vi "laneleftright4_2_1.vi"() -> (2 "Coeff right":dbl[](array[numeric]), 3 "Coeff left":dbl[](array[numeric]))   [LabVIEW 2015]
uses:
  <vilib>/Analysis/polynomials.llb/Remove Zero Threshold Type.ctl
  G_SEN.vi
  <vilib>/Analysis/1siggen.llb/Ramp Pattern by Delta.vi
  G_LCM.vi
  <vilib>/Analysis/polynomials.llb/1D Polynomial Evaluation (DBL).vi
  <vilib>/Analysis/polynomials.llb/Remove Zero Coefficients (DBL).vi
  G_ALL.vi
  <vilib>/Analysis/NI_AALPro.lvlib
  <vilib>/Analysis/NI_AALBase.lvlib
  <vilib>/gmath/NI_Gmath.lvlib
panel:
  out "stop_shift":dbl
  in  "y 4":dbl
  in  "y 3":dbl
  out "f":dbl
  out "x0, y0, z0 2":dbl[](array[numeric]) format="%.2f"
  out "r":dbl format="%.2f"
  in  "threshold":dbl
  out "y 2":dbl[](array[numeric])
  out "x 2":dbl[](array[numeric])
  out "w 2":dbl[](array[numeric])
  out "lane_right_pt":dbl[][](array[numeric])
  in  "x_gain":dbl=1.0 min=-1.0 max=1.0
  in  "y_gain":dbl=1.0 min=-1.0 max=1.0
  out "map_track 2":dbl[][](array[numeric])
  in  "d_safe":dbl=1.1 format="%#_13g"
  out "map_track":dbl[][](array[numeric])
  out "lane_left_pt":dbl[][](array[numeric])
  out "x_shift":dbl format="%#_13g"
  out "y_shift":dbl format="%#_13g"
  in  "lane_gain":dbl=0.7 min=-1.0 max=1.0
  out "Lane_C_M":dbl[](array[numeric])=[0.8601491478953653, 0.8717844136967624, 0.882947592858927, 0.8936326403234123, 0.9038337699485205, 0.9135454576426009, 0.9227624443554423, 0.9314797389261423, 0.9396926207859084, 0.9473966425143293, 0.9545876322477319, 0.9612616959383189, 0.9674152194628639, 0.9730448705798238, 0.9781476007338057, 0.9827206467064133, 0.9867615321125792, 0.9902680687415704, 0.993238357741943, 0.9956707906498045, 0.9975640502598242, 0.9989171113385246, 0.9997292411794617, 1.0, 0.9997292411794617, 0.9989171113385246, 0.9975640502598242, 0.9956707906498045, 0.993238357741943, 0.9902680687415704, 0.9867615321125792, 0.9827206467064133]
  out "ratio(-1:left1:right)":dbl
  out "NaN/Path/Refnum?":bool
  out "Rleft":dbl
  out "Rright":dbl
  in  "poly":i32=2 min=1 max=5 step=1
  out "Coeff stop":dbl[](array[numeric])
  out "y_end":dbl[](array[numeric])=[0.8601491478953653, 0.8717844136967624, 0.882947592858927, 0.8936326403234123, 0.9038337699485205, 0.9135454576426009, 0.9227624443554423, 0.9314797389261423, 0.9396926207859084, 0.9473966425143293, 0.9545876322477319, 0.9612616959383189, 0.9674152194628639, 0.9730448705798238, 0.9781476007338057, 0.9827206467064133, 0.9867615321125792, 0.9902680687415704, 0.993238357741943, 0.9956707906498045, 0.9975640502598242, 0.9989171113385246, 0.9997292411794617, 1.0, 0.9997292411794617, 0.9989171113385246, 0.9975640502598242, 0.9956707906498045, 0.993238357741943, 0.9902680687415704, 0.9867615321125792, 0.9827206467064133]
  in  "iter":i32=7
  out "Waveform Graph":dbl[](graph)
  out "w":dbl[](array[numeric])
  out "XY Graph 4":cluster{"Y":dbl[], "Y":dbl[]}[](graph)=[{"Y"=array[3210 elements], "Y"=array[3210 elements]}, {"Y"=[-0.0, 0.001154394197769193, 0.004617650635850623, 0.010389990872226917, 0.018471784248973222, 0.02886354801042046, 0.041565947468740205, 0.056579796217107514, 0.0739060563904701, 0.0935458389742223, 0.11550040416098284, 0.13977116175580306, 0.16635967162997645, 0.19526764422393228, 0.2264969410994837, 0.26004957554195585, 0.2959277132125635, 0.3341336728515216, 0.374669927032528, 0.417539102969144, 0.4627439833735707, 0.5102875073687159, 0.560172771454063, 0.6124030305261954, 0.6669816989546717, 0.7239123517142048, 0.7831987255740245, 0.8448447203451934, 0.9088544001870815, 0.975231994973953, 1.0439819017227023, 1.1151086860829622, 1.1886170838907617, 1.2645120027869723, 1.342798523901962, 1.42348190360768, 1.5065675753387922, 1.592061151484188, 1.6799684253507792, 1.770295373200753, 1.8630481563645134, 1.9582331234307588, 2.0558568125157564, 2.1559259536137603, 2.258447471030621], "Y"=[0.0, 0.5, 1.0, 1.5, 2.0, 2.5, 3.0, 3.5, 4.0, 4.5, 5.0, 5.5, 6.0, 6.5, 7.0, 7.5, 8.0, 8.5, 9.0, 9.5, 10.0, 10.5, 11.0, 11.5, 12.0, 12.5, 13.0, 13.5, 14.0, 14.5, 15.0, 15.5, 16.0, 16.5, 17.0, 17.5, 18.0, 18.5, 19.0, 19.5, 20.0, 20.5, 21.0, 21.5, 22.0]}, {"Y"=[0.362252581831572], "Y"=[-0.8199241909738847]}, {"Y"=array[210 elements], "Y"=array[210 elements]}, {"Y"=[-0.925, -0.925, -0.925, -0.6775, -0.6775, -0.925, -0.925, -0.925, -0.925, -0.6775, -0.6775, -0.925, -0.925, -0.925, 0.9025, 0.9025, 0.9025, 0.6775, 0.6775, 0.9025, 0.9025, 0.9025, 0.9025, 0.6775, 0.6775, 0.9025, 0.9025, 0.9025, -0.925], "Y"=[-0.75, -0.224, 0.224, 0.224, -0.224, -0.224, 0.224, 2.415, 2.885, 2.885, 2.415, 2.415, 2.885, 3.5, 3.5, 2.885, 2.415, 2.415, 2.885, 2.885, 2.415, 0.224, -0.224, -0.224, 0.224, 0.224, -0.224, -0.75, -0.75]}, {"Y"=[0.171875, 0.15377271904051304, 0.1346290179491043, 0.11445423440635205, 0.09325870609283447, 0.07105277068912982, 0.04784676587581635, 0.02365102933347224, -0.0015241012573242174, -0.02766828821599482, -0.05477119386196136, -0.08282248051464558, -0.11181181049346922, -0.14172884611785413, -0.17256324970722198, -0.20430468358099463, -0.23694281005859374, -0.27046729145944115, -0.30486779010295867, -0.340133968308568, -0.3762554883956909, -0.41322201268374914, -0.4510232034921646, -0.4896487231403589], "Y"=[0.0, 0.5, 1.0, 1.5, 2.0, 2.5, 3.0, 3.5, 4.0, 4.5, 5.0, 5.5, 6.0, 6.5, 7.0, 7.5, 8.0, 8.5, 9.0, 9.5, 10.0, 10.5, 11.0, 11.5]}, {"Y"=[1.796875, 1.778772719040513, 1.7596290179491043, 1.739454234406352, 1.7182587060928345, 1.6960527706891297, 1.6728467658758164, 1.6486510293334722, 1.6234758987426758, 1.5973317117840051, 1.5702288061380387, 1.5421775194853544, 1.513188189506531, 1.483271153882146, 1.452436750292778, 1.4206953164190055, 1.3880571899414063, 1.354532708540559, 1.3201322098970414, 1.284866031691432, 1.248744511604309, 1.2117779873162509, 1.1739767965078354, 1.135351276859641, 1.0959117660522462, 1.0556686017662287, 1.014632121682167, 0.9728126634806396, 0.9302205648422242, 0.8868661634474992], "Y"=[0.0, 0.5, 1.0, 1.5, 2.0, 2.5, 3.0, 3.5, 4.0, 4.5, 5.0, 5.5, 6.0, 6.5, 7.0, 7.5, 8.0, 8.5, 9.0, 9.5, 10.0, 10.5, 11.0, 11.5, 12.0, 12.5, 13.0, 13.5, 14.0, 14.5]}, {"Y"=[-1.453125, -1.471227280959487, -1.4903709820508957, -1.510545765593648, -1.5317412939071655, -1.5539472293108703, -1.5771532341241836, -1.6013489706665278, -1.6265241012573242, -1.6526682882159949, -1.6797711938619613, -1.7078224805146456, -1.736811810493469, -1.766728846117854, -1.797563249707222, -1.8293046835809945, -1.8619428100585937, -1.895467291459441, -1.9298677901029586], "Y"=[0.0, 0.5, 1.0, 1.5, 2.0, 2.5, 3.0, 3.5, 4.0, 4.5, 5.0, 5.5, 6.0, 6.5, 7.0, 7.5, 8.0, 8.5, 9.0]}, {"Y"=[0.171875, 0.2568230007600336, 0.3384052130063493, 0.44574342526006827, 0.5205081969556753, 0.5917680690742042, 0.659409530134929, 0.7229937549325056, 0.7835496148685115, 0.8405449546633443, 0.9258576868463875], "Y"=[-20.239964538708662, -19.725637940364884, -19.211158961966362, -18.6998967366845, -18.19022720070031, -17.681887266143153, -17.17615515566314, -16.67683575591291, -16.176265245349786, -15.679082775270938, -15.183754484614711]}, {"Y"=[7.134647485270904], "Y"=[38.71960961082238]}, {"Y"=array[980 elements], "Y"=array[980 elements]}, {"Y"=[], "Y"=[]}]
  out "y":dbl[](array[numeric])
  out "x":dbl[](array[numeric])
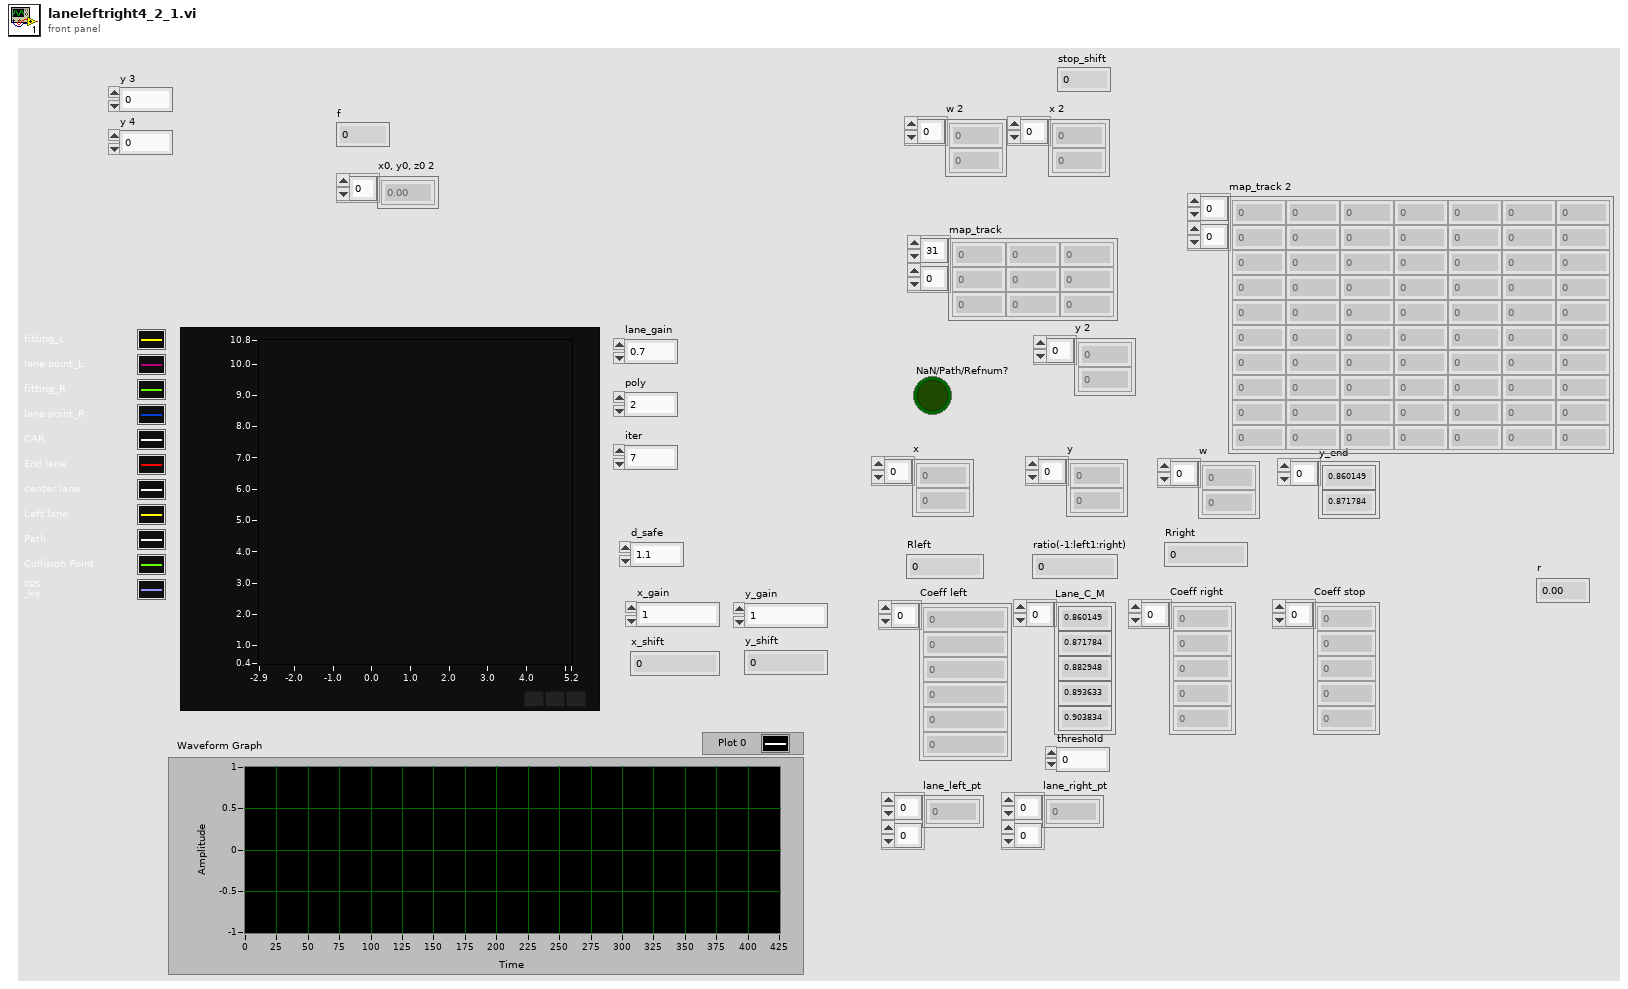
[diagram p1: front panel]
types:
  T1 = cluster{"hash":i64, "sys time":i64, "size":i64, "x":dbl[], "y":dbl[], "point_flag":i32[]}
  T2 = cluster{"delta":bool, "Rotational position":dbl, "Rotational position":dbl}[]
  T3 = typedef "NI_AALPro.lvlib/Remove Zero Threshold Type.ctl" = u16
  T4 = cluster{"C_Wheel base":dbl, "ratio_steer":dbl, "Overall width":dbl, "af":dbl, "turn radius":dbl, "eval":dbl, "ap":dbl, "an":dbl, "Vmax":dbl, "mu":dbl, "Vlast":dbl}
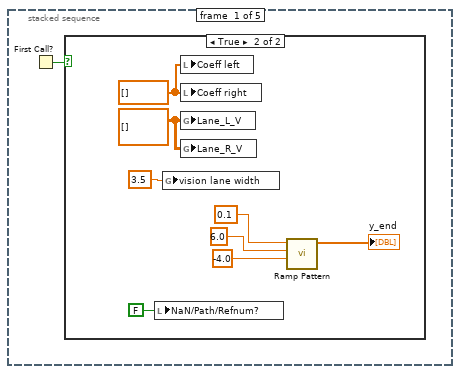
[diagram p2: hidden frame]
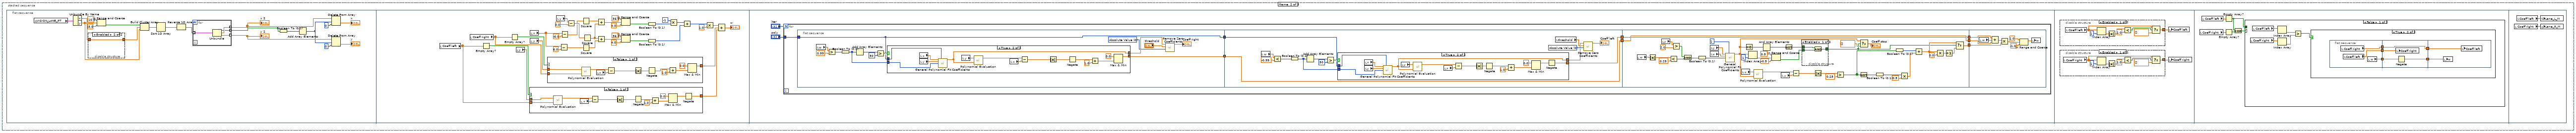
[diagram p4: hidden frame]
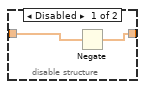
[diagram p5: hidden frame]
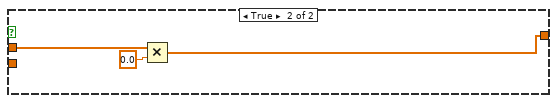
[diagram p6: hidden frame]
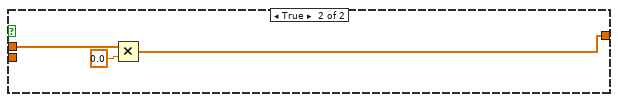
[diagram p7: hidden frame]
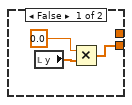
[diagram p8: hidden frame]
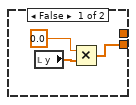
[diagram p9: hidden frame]
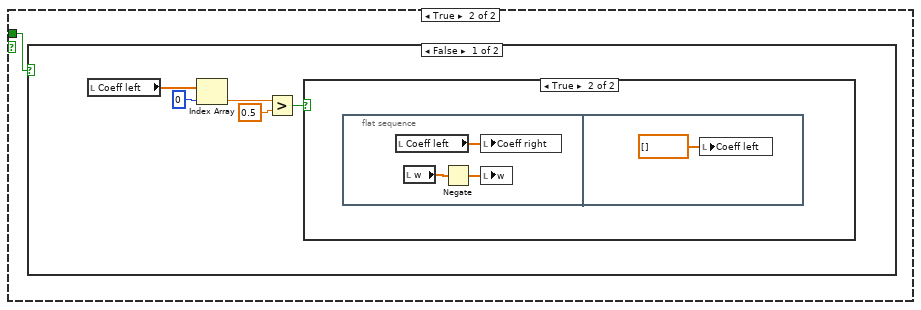
[diagram p14: hidden frame]
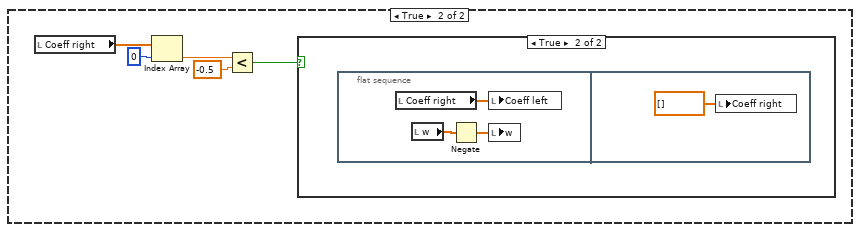
[diagram p16: hidden frame]
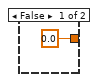
[diagram p19: hidden frame]
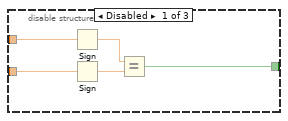
[diagram p20: hidden frame]
diagram:
  n1 = stacked-sequence {
    frame #0 {
      n2 = First Call?() -> (First Call?: T/F=w1:bool)
      n3 = case shown="True" w1 {
        frame False {
        }
        frame True {
          w2 = dbl[] [] ("Coeff left")
          w4 = dbl[][] [] ("Lane_R_V")
          n4 = local write "NaN/Path/Refnum?"(FALSE ("NaN/Path/Refnum?")) -> ()
          n5 = global write "G_SEN.vi" "vision lane width"(3.5 ("vision lane width")) -> ()
          n6 = local write "Coeff left"(w2) -> ()
          n7 = local write "Coeff right"(w2) -> ()
          n8 = global write "G_SEN.vi" "Lane_L_V"(w4) -> ()
          n9 = global write "G_SEN.vi" "Lane_R_V"(w4) -> ()
          n10 = call-poly <vilib>:"Ramp Pattern.vi"("start"=-4.0, "end"=6.0, "delta"=0.1) -> ("Ramp Pattern"=→"y_end":dbl[])  [unwired: 6 in, 2 out]
        }
      }
    }
    frame #1 {
      n11 = flat-sequence {
        frame #0 {
          n12 = global read "G_LCM.vi" "VISION_LANE_PT"() -> (w12:T1)
          n13 = Unbundle By Name(w12) -> ("x"=w27:dbl[], "y"=w21:dbl[])
          n14 = disable-structure shown="Enabled" {
            disable-tunnel: w27 -> [w30 w31]
            disable-tunnel: [w29 w31] -> w28
            frame Disabled {
              n15 = Negate(x=w30) -> (-x=w29:dbl[])
            }
            frame Enabled {
            }
          }
          n16 = In Range and Coerce(upper limit=10.0 ("delta"), x=w21, lower limit=-3.0) -> (In Range?=w19:bool[])  [unwired: 1 out]
          n17 = Build Cluster Array(w19, w28, w21) -> (w17:T2)
          n18 = Sort 1D Array(array=w17) -> (sorted array=w18:T2)
          n19 = Reverse 1D Array(array=w18) -> (reversed array=w14:T2)
          n20 = for {
            tunnel: w14 -> [w35] mode=indexing
            tunnel: [w34] -> w11 mode=indexing
            tunnel: [w33] -> w10 mode=indexing
            tunnel: [w32] -> w22 mode=indexing
            n21 = Unbundle(w35) -> ("delta"=w32:bool, "Rotational position"=w34:dbl, "Rotational position"=w33:dbl)
          }
          "x 2" <- w11
          "y 2" <- w10
          n22 = Boolean To (0,1)(Boolean=w22) -> (0, 1=w15:i16[])
          n23 = Add Array Elements(numeric array=w15) -> (sum=w23:i16)
          n24 = Delete From Array(array=w11, length=w23, index=0) -> (deleted portion=→"x":dbl[])  [unwired: 1 out]
          n25 = Delete From Array(array=w10, length=w23, index=0) -> (deleted portion=→"y":dbl[])  [unwired: 1 out]
        }
        frame #1 {
          n26 = local read "Coeff left"() -> (w67:dbl[])
          n27 = local read "Coeff right"() -> (w66:dbl[])
          n28 = Empty Array?(array=w67) -> (empty?=w68:bool)
          n29 = Empty Array?(array=w66) -> (empty?=w69:bool)
          n30 = local read "y"() -> (w64:dbl[])
          n31 = case shown="False" w68 {
            tunnel: w64 -> [w90 w98]
            tunnel: w67 -> [w87 _]
            tunnel: [w85 w97] -> w65
            frame False {
              n32 = call-poly <vilib>:"Polynomial Evaluation.vi"("P(x)"=w87, "A"=w90) -> ("P(A)"=w89:dbl[])  [unwired: 1 out]
              n33 = local read "x"() -> (w88:dbl[])
              n34 = Subtract(x=w89, y=w88) -> (x-y=w94:dbl[])
              n35 = Absolute Value(x=w94) -> (abs(x)=w93:dbl[])
              n36 = Negate(x=w93) -> (-x=w92:dbl[])
              n37 = Add(x=w92, y=1.0) -> (x+y=w96:dbl[])
              n38 = Max & Min(x=0.0, y=w96) -> (max(x,y)=w86:dbl[])  [unwired: 1 out]
              n39 = Negate(x=w86) -> (-x=w85:dbl[])
            }
            frame True {
              n40 = Multiply(x=w98, y=0.0) -> (x*y=w97:dbl[])
            }
          }
          n41 = local read "x"() -> (w36:dbl[])
          n42 = local read "y"() -> (w70:dbl[])
          n43 = case shown="False" w69 {
            tunnel: [w79 w82] -> w62
            tunnel: w66 -> [w78 _]
            tunnel: w70 -> [w71 w83]
            frame False {
              n44 = call-poly <vilib>:"Polynomial Evaluation.vi"("P(x)"=w78, "A"=w71) -> ("P(A)"=w76:dbl[])  [unwired: 1 out]
              n45 = local read "x"() -> (w77:dbl[])
              n46 = Subtract(x=w76, y=w77) -> (x-y=w72:dbl[])
              n47 = Absolute Value(x=w72) -> (abs(x)=w73:dbl[])
              n48 = Negate(x=w73) -> (-x=w74:dbl[])
              n49 = Add(x=w74, y=1.0) -> (x+y=w80:dbl[])
              n50 = Max & Min(x=0.0, y=w80) -> (max(x,y)=w79:dbl[])  [unwired: 1 out]
            }
            frame True {
              n51 = Multiply(x=w83, y=0.0) -> (x*y=w82:dbl[])
            }
          }
          n52 = local read "y"() -> (w37:dbl[])
          n53 = Subtract(x=w36, y=6.0) -> (x-y=w40:dbl[])
          n54 = Subtract(x=w36, y=-6.0) -> (x-y=w42:dbl[])
          n55 = Subtract(x=w37, y=0.0) -> (x-y=w49:dbl[])
          n56 = Square(x=w42) -> (x^2=w41:dbl[])
          n57 = Square(x=w40) -> (x^2=w50:dbl[])
          n58 = Square(x=w49) -> (x^2=w51:dbl[])
          n59 = Add(x=w41, y=w51) -> (x+y=w57:dbl[])
          n60 = Add(x=w51, y=w50) -> (x+y=w52:dbl[])
          n61 = In Range and Coerce(upper limit=36.0, x=w57, lower limit=4.0) -> (In Range?=w59:bool[])  [unwired: 1 out]
          n62 = In Range and Coerce(upper limit=36.0, x=w52, lower limit=4.0) -> (In Range?=w58:bool[])  [unwired: 1 out]
          n63 = Boolean To (0,1)(Boolean=w59) -> (0, 1=w60:i16[])
          n64 = Boolean To (0,1)(Boolean=w58) -> (0, 1=w61:i16[])
          n65 = Multiply(x=i16 -1, y=w60) -> (x*y=w45:i16[])
          n66 = Add(x=w45, y=w61) -> (x+y=w47:i16[])
          n67 = Multiply(x=w47, y=1.0 ("element")) -> (x*y=w63:dbl[])
          n68 = Compound Arithmetic op=ADD(w63, w62, w65) -> (→"w":dbl[])
        }
        frame #2 {
          n69 = for {
            N: "iter" -> [_]
            tunnel: "poly" -> [w103]
            n70 = flat-sequence {
              tunnel: [w120] -> w109
              tunnel: w103 -> [w114]
              tunnel: [w114] -> w102
              tunnel: [w154] -> w108
              tunnel: w109 -> [w154]
              tunnel: [w151] -> w106
              tunnel: w102 -> [w145]
              tunnel: w108 -> [w216]
              tunnel: [w216] -> w107
              tunnel: w106 -> [w215]
              tunnel: [w215] -> w105
              tunnel: [w186] -> w104
              tunnel: w107 -> [w224]
              tunnel: w105 -> [w220]
              tunnel: w104 -> [w222]
              frame #0 {
                w113 = T3 0 items=["Absolute Value", "Relative Value"] ("threshold type")
                n71 = local read "w"() -> (w122:dbl[])
                n72 = Greater?(x=w122, y=0.99) -> (0:w115:bool[])
                n73 = Boolean To (0,1)(Boolean=w115) -> (0, 1=w116:i16[])
                n74 = Add Array Elements(numeric array=w116) -> (sum=w119:i16)
                n75 = Greater?(x=w119, y=i16 50) -> (0:w117:bool)
                n76 = case shown="True" w117 {
                  tunnel: [w124 w131] -> w120
                  tunnel: [_ w130] -> w112
                  tunnel: w116 -> [_ w127]
                  tunnel: w114 -> [_ w126]
                  frame False {
                    n77 = local read "y"() -> (w125:dbl[])
                    n78 = Multiply(x=0.0, y=w125) -> (x*y=w124:dbl[])
                  }
                  frame True {
                    n79 = local read "x"() -> (w128:dbl[])
                    n80 = local read "y"() -> (w129:dbl[])
                    n81 = call <vilib>:"General Polynomial Fit Coefficients.vi"("Y"=w128, "polynomial order"=w126, "X"=w129, "Weight"=w127) -> ("Polynomial Coefficients"=w130:dbl[])  [unwired: 10 in, 1 out]
                    n82 = local read "y"() -> (w140:dbl[])
                    n83 = call-poly <vilib>:"Polynomial Evaluation.vi"("P(x)"=w130, "A"=w140) -> ("P(A)"=w139:dbl[])  [unwired: 1 out]
                    n84 = local read "x"() -> (w138:dbl[])
                    n85 = Subtract(x=w139, y=w138) -> (x-y=w137:dbl[])
                    n86 = Absolute Value(x=w137) -> (abs(x)=w136:dbl[])
                    n87 = Negate(x=w136) -> (-x=w135:dbl[])
                    n88 = Add(x=w135, y=1.0) -> (x+y=w132:dbl[])
                    n89 = Max & Min(x=0.0, y=w132) -> (max(x,y)=w131:dbl[])  [unwired: 1 out]
                  }
                }
                n90 = call-poly <vilib>:"Remove Zero Coefficients.vi"("threshold type"=w113, "threshold"="threshold", "P(x) In"=w112) -> ("P(x) Out"=→"Coeff right":dbl[])  [unwired: 6 in, 2 out]
              }
              frame #1 {
                w144 = T3 0 items=["Absolute Value", "Relative Value"] ("threshold type")
                n91 = local read "w"() -> (w152:dbl[])
                n92 = Less?(x=w152, y=-0.99) -> (x < y?=w148:bool[])
                n93 = Boolean To (0,1)(Boolean=w148) -> (0, 1=w146:i16[])
                n94 = Add Array Elements(numeric array=w146) -> (sum=w149:i16)
                n95 = Greater?(x=w149, y=i16 50) -> (0:w147:bool)
                n96 = case shown="True" w147 {
                  tunnel: [w155 w163] -> w151
                  tunnel: [_ w162] -> w143
                  tunnel: w146 -> [_ w159]
                  tunnel: w145 -> [_ w158]
                  frame False {
                    n97 = local read "y"() -> (w156:dbl[])
                    n98 = Multiply(x=0.0, y=w156) -> (x*y=w155:dbl[])
                  }
                  frame True {
                    n99 = local read "x"() -> (w160:dbl[])
                    n100 = local read "y"() -> (w161:dbl[])
                    n101 = call <vilib>:"General Polynomial Fit Coefficients.vi"("Y"=w160, "polynomial order"=w158, "X"=w161, "Weight"=w159) -> ("Polynomial Coefficients"=w162:dbl[])  [unwired: 10 in, 1 out]
                    n102 = local read "y"() -> (w167:dbl[])
                    n103 = call-poly <vilib>:"Polynomial Evaluation.vi"("P(x)"=w162, "A"=w167) -> ("P(A)"=w168:dbl[])  [unwired: 1 out]
                    n104 = local read "x"() -> (w169:dbl[])
                    n105 = Subtract(x=w168, y=w169) -> (x-y=w170:dbl[])
                    n106 = Absolute Value(x=w170) -> (abs(x)=w171:dbl[])
                    n107 = Negate(x=w171) -> (-x=w165:dbl[])
                    n108 = Add(x=w165, y=1.0) -> (x+y=w172:dbl[])
                    n109 = Max & Min(x=0.0, y=w172) -> (max(x,y)=w166:dbl[])  [unwired: 1 out]
                    n110 = Negate(x=w166) -> (-x=w163:dbl[])
                  }
                }
                n111 = local read "threshold"() -> (w141:dbl)
                n112 = call-poly <vilib>:"Remove Zero Coefficients.vi"("threshold type"=w144, "threshold"=w141, "P(x) In"=w143) -> ("P(x) Out"=→"Coeff left":dbl[])  [unwired: 6 in, 2 out]
              }
              frame #2 {
                n113 = local read "w"() -> (w194:dbl[])
                n114 = Absolute Value(x=w194) -> (abs(x)=w193:dbl[])
                n115 = local read "y"() -> (w198:dbl[])
                n116 = Less?(x=w193, y=0.25) -> (x < y?=w192:bool[])
                n117 = Greater?(x=w198, y=2.0) -> (0:w196:bool[])
                n118 = And(x=w196, y=w192) -> (x .and. y?=w195:bool[])
                n119 = Boolean To (0,1)(Boolean=w195) -> (0, 1=w214:i16[])
                n120 = local read "y"() -> (w208:dbl[])
                n121 = local read "x"() -> (w207:dbl[])
                n122 = call <vilib>:"General Polynomial Fit Coefficients.vi"("Y"=w208, "polynomial order"=1, "X"=w207, "Weight"=w214) -> ("Polynomial Coefficients"=w179:dbl[])  [unwired: 10 in, 1 out]
                n123 = local read "x"() -> (w212:dbl[])
                n124 = Equal To 0?(x=w179) -> (x = 0?=w178:bool[])
                n125 = Index Array(array=w179, index=1) -> (element=w189:dbl)
                n126 = call-poly <vilib>:"Polynomial Evaluation.vi"("P(x)"=w179, "A"=w212) -> ("P(A)"=w211:dbl[])  [unwired: 1 out]
                n127 = And Array Elements(Boolean array=w178) -> (logical AND=w175:bool)
                n128 = In Range and Coerce(upper limit=0.5, x=w189, lower limit=-0.5) -> (In Range?=w177:bool)  [unwired: 1 out]
                n129 = local read "y"() -> (w210:dbl[])
                n130 = Not(x=w175) -> (.not. x?=w174:bool)
                n131 = Subtract(x=w211, y=w210) -> (x-y=w209:dbl[])
                n132 = disable-structure shown="Enabled" {
                  disable-tunnel: w177 -> [w219 _]
                  disable-tunnel: [w218 _] -> w176
                  disable-tunnel: w174 -> [w217 _]
                  frame Enabled {
                    n133 = And(x=w217, y=w219) -> (x .and. y?=w218:bool)
                  }
                  frame Disabled {
                  }
                }
                n134 = Absolute Value(x=w209) -> (abs(x)=w206:dbl[])
                n135 = Greater?(x=w206, y=0.25 ("Numeric 2")) -> (0:w204:bool[])
                n136 = Not(x=w204) -> (.not. x?=w203:bool[])
                n137 = Select(t=w179, s=w176, f=dbl[] []) -> (s? t:f=→"Coeff stop":dbl[])
                n138 = Boolean To (0,1)(Boolean=w203) -> (0, 1=w202:i16[])
                n139 = Boolean To (0,1)(Boolean=w204) -> (0, 1=w199:i16[])
                n140 = Multiply(x=w202, y=0.5) -> (x*y=w200:dbl[])
                n141 = Add(x=w199, y=w200) -> (x+y=w185:dbl[])
                n142 = Multiply(x=w185, y=0.0) -> (x*y=w183:dbl[])
                n143 = Increment(x=w183) -> (x+1=w182:dbl[])
                n144 = Select(t=w185, s=w176, f=w182) -> (s? t:f=w186:dbl[])
              }
              frame #3 {
                n145 = local read "w"() -> (w228:dbl[])
                n146 = Compound Arithmetic op=ADD(w220, w228, w224) -> (w221:dbl[])
                n147 = Multiply(x=w221, y=w222) -> (x*y=w223:dbl[])
                n148 = In Range and Coerce(upper limit=1.0, x=w223, lower limit=-1.0) -> (coerced(x)=w225:dbl[])  [unwired: 1 out]
                n149 = local write "w"(w225) -> ()
              }
            }
          }
        }
        frame #3 {
          n150 = disable-structure shown="Enabled" {
            disable-tunnel: [w232 _] -> w229
            frame Enabled {
              n151 = local read "Coeff left"() -> (w231:dbl[])
              n152 = Index Array(array=w231, index=1) -> (element=w234:dbl)
              n153 = Absolute Value(x=w234) -> (abs(x)=w235:dbl)
              n154 = Less?(x=w235, y=1.0) -> (x < y?=w237:bool)
              n155 = Select(t=w231, s=w237, f=dbl[] []) -> (s? t:f=w232:dbl[])
            }
            frame Disabled {
            }
          }
          n156 = disable-structure shown="Enabled" {
            disable-tunnel: [w241 _] -> w230
            frame Enabled {
              n157 = local read "Coeff right"() -> (w239:dbl[])
              n158 = Index Array(array=w239, index=1) -> (element=w245:dbl)
              n159 = Absolute Value(x=w245) -> (abs(x)=w244:dbl)
              n160 = Less?(x=w244, y=1.0) -> (x < y?=w242:bool)
              n161 = Select(t=w239, s=w242, f=dbl[] []) -> (s? t:f=w241:dbl[])
            }
            frame Disabled {
            }
          }
          n162 = local write "Coeff left"(w229) -> ()
          n163 = local write "Coeff right"(w230) -> ()
        }
        frame #4 {
          n164 = local read "Coeff right"() -> (w248:dbl[])
          n165 = local read "Coeff left"() -> (w247:dbl[])
          n166 = Empty Array?(array=w247) -> (empty?=w251:bool)
          n167 = Empty Array?(array=w248) -> (empty?=w249:bool)
          n168 = Exclusive Or(1:w249, 2:w251) -> (0:w250:bool)
          n169 = case shown="False" w250 {
            tunnel: w251 -> [_ w271]
            frame False {
              n170 = local read "Coeff right"() -> (w255:dbl[])
              n171 = local read "Coeff left"() -> (w256:dbl[])
              n172 = Index Array(array=w256) -> (element=w254:dbl)  [unwired: 1 in]
              n173 = Index Array(array=w255) -> (element=w253:dbl)  [unwired: 1 in]
              n174 = Greater?(x=w254, y=w253) -> (0:w252:bool)
              n175 = case shown="True" w252 {
                frame False {
                }
                frame True {
                  n176 = flat-sequence {
                    tunnel: [w264] -> w260
                    tunnel: [w263] -> w259
                    tunnel: [w262] -> w258
                    tunnel: [w268] -> w261
                    tunnel: w260 -> [w268]
                    tunnel: w259 -> [w267]
                    tunnel: w258 -> [w266]
                    tunnel: [w265] -> w257
                    tunnel: w261 -> [w270]
                    tunnel: w257 -> [w269]
                    frame #0 {
                      n177 = local read "Coeff right"() -> (w264:dbl[])
                      n178 = local read "Coeff left"() -> (w263:dbl[])
                      n179 = local read "w"() -> (w262:dbl[])
                    }
                    frame #1 {
                      n180 = local write "Coeff right"(w267) -> ()
                      n181 = Negate(x=w266) -> (-x=w265:dbl[])
                    }
                    frame #2 {
                      n182 = local write "w"(w269) -> ()
                      n183 = local write "Coeff left"(w270) -> ()
                    }
                  }
                }
              }
            }
            frame True {
              n184 = case shown="False" w271 {
                frame False {
                  n185 = local read "Coeff left"() -> (w276:dbl[])
                  n186 = Index Array(array=w276, index=0) -> (element=w274:dbl)
                  n187 = Greater?(x=w274, y=0.5) -> (0:w272:bool)
                  n188 = case shown="True" w272 {
                    frame False {
                    }
                    frame True {
                      n189 = flat-sequence {
                        frame #0 {
                          n190 = local read "Coeff left"() -> (w279:dbl[])
                          n191 = local read "w"() -> (w278:dbl[])
                          n192 = Negate(x=w278) -> (-x=w277:dbl[])
                          n193 = local write "Coeff right"(w279) -> ()
                          n194 = local write "w"(w277) -> ()
                        }
                        frame #1 {
                          n195 = local write "Coeff left"(dbl[] []) -> ()
                        }
                      }
                    }
                  }
                }
                frame True {
                  n196 = local read "Coeff right"() -> (w285:dbl[])
                  n197 = Index Array(array=w285, index=0) -> (element=w283:dbl)
                  n198 = Less?(x=w283, y=-0.5) -> (x < y?=w281:bool)
                  n199 = case shown="True" w281 {
                    frame False {
                    }
                    frame True {
                      n200 = flat-sequence {
                        frame #0 {
                          n201 = local read "Coeff right"() -> (w288:dbl[])
                          n202 = local read "w"() -> (w287:dbl[])
                          n203 = Negate(x=w287) -> (-x=w286:dbl[])
                          n204 = local write "Coeff left"(w288) -> ()
                          n205 = local write "w"(w286) -> ()
                        }
                        frame #1 {
                          n206 = local write "Coeff right"(dbl[] []) -> ()
                        }
                      }
                    }
                  }
                }
              }
            }
          }
        }
        frame #5 {
          n207 = local read "Coeff right"() -> (w290:dbl[])
          n208 = local read "Coeff left"() -> (w291:dbl[])
          n209 = global write "G_SEN.vi" "Lane_L_M"(w291) -> ()
          n210 = global write "G_SEN.vi" "Lane_R_M"(w290) -> ()
        }
      }
    }
    frame #2 {
      n211 = flat-sequence {
        frame #0 {
          n212 = local read "Coeff right"() -> (w293:dbl[])
          n213 = local read "Coeff right"() -> (w321:dbl[])
          n214 = local read "Coeff left"() -> (w292:dbl[])
          n215 = local read "Coeff left"() -> (w319:dbl[])
          n216 = Empty Array?(array=w292) -> (empty?=w295:bool)
          n217 = Empty Array?(array=w293) -> (empty?=w296:bool)
          n218 = Empty Array?(array=w321) -> (empty?=w315:bool)
          n219 = Empty Array?(array=w319) -> (empty?=w313:bool)
          n220 = Index Array(array=w321, index #1=1 ("index")) -> (element #1=w297:dbl, element #2=w304:dbl)  [unwired: 1 in]
          n221 = Index Array(array=w319, index #1=1 ("index")) -> (element #1=w312:dbl, element #2=w305:dbl)  [unwired: 1 in]
          n222 = Or(x=w295, y=w296) -> (x .or. y?=w294:bool)
          n223 = Square(x=w297) -> (x^2=w298:dbl)
          n224 = Square(x=w312) -> (x^2=w311:dbl)
          n225 = case shown="False" w294 {
            frame False {
              n226 = local read "Coeff right"() -> (w328:dbl[])
              n227 = local read "Coeff left"() -> (w325:dbl[])
              n228 = Subtract(x=w328, y=w325) -> (x-y=w326:dbl[])
              n229 = Index Array(array=w326, index=0) -> (element=w329:dbl)
              n230 = Max & Min(x=w329, y=2.0) -> (max(x,y)=w330:dbl)  [unwired: 1 out]
              n231 = global write "G_SEN.vi" "vision lane width"(w330) -> ()
            }
            frame True {
            }
          }
          n232 = Increment(x=w298) -> (x+1=w300:dbl)
          n233 = Increment(x=w311) -> (x+1=w309:dbl)
          n234 = Multiply(x=w304, y=2.0) -> (x*y=w302:dbl)
          n235 = Square Root(x=w300) -> (sqrt(x)=w299:dbl)
          n236 = Square Root(x=w309) -> (sqrt(x)=w310:dbl)
          n237 = Multiply(x=w305, y=2.0) -> (x*y=w307:dbl)
          n238 = Multiply(x=w299, y=w300) -> (x*y=w301:dbl)
          n239 = Multiply(x=w310, y=w309) -> (x*y=w308:dbl)
          n240 = Divide(x=w301, y=w302) -> (x/y=w316:dbl)
          n241 = Divide(x=w308, y=w307) -> (x/y=w314:dbl)
          n242 = Select(t=inf, s=w315, f=w316) -> (s? t:f=→"Rright":dbl)
          n243 = Select(t=inf, s=w313, f=w314) -> (s? t:f=→"Rleft":dbl)
        }
        frame #1 {
          n244 = global read "G_ALL.vi" "map_track 2"() -> (w361:dbl[][])
          n245 = Array Subset(array=w361, index (row)=40 ("index"), length (row)=10 ("length")) -> (w357:dbl[][])  [unwired: 2 in]
          n246 = Array Subset(array=w361, index (row)=29 ("index"), length (row)=3 ("length")) -> (w358:dbl[][])  [unwired: 2 in]
          n247 = Index Array(array=w357, index (col) #1=0 ("disabled index (col)")) -> (element #1=w353:dbl[], element #2=w347:dbl[])  [unwired: 3 in]
          n248 = Index Array(array=w358, index (col) #1=0 ("disabled index (col)")) -> (element #1=w352:dbl[], element #2=w354:dbl[])  [unwired: 3 in]
          n249 = Array Size(array=w347) -> (size(s)=w346:i32)
          n250 = Array Size(array=w352) -> (size(s)=w349:i32)
          n251 = Initialize Array(0 ("dimension size"), w346) -> (w345:i32[])
          n252 = Initialize Array(0 ("dimension size"), w349) -> (w351:i32[])
          n253 = call <vilib>:"Fitting on a Sphere.vi"("Z"=w345, "Y"=w347, "X"=w353) -> ("r"=w343:dbl, "x0, y0, z0"=w336:dbl[])  [unwired: 1 out]
          "x0, y0, z0 2" <- w336
          n254 = call <vilib>:"Fitting on a Sphere.vi"("Z"=w351, "Y"=w354, "X"=w352) -> ("r"=w344:dbl)  [unwired: 2 out]
          "r" <- w344
          n255 = Index Array(array=w336, index=0) -> (element=w335:dbl)
          n256 = Greater?(x=w344, y="y 3") -> (0:w342:bool)
          n257 = Less?(x=w343, y="y 4") -> (x < y?=w341:bool)
          n258 = And(x=w342, y=w341) -> (x .and. y?=w338:bool)
          n259 = Greater?(x=w335, y=0.0) -> (0:w337:bool)
          n260 = case shown="True" w338 {
            tunnel: w337 -> [_ w365]
            tunnel: [0.0 ("f") w366] -> w334
            frame False {
            }
            frame True {
              n261 = Select(t=-0.3, s=w365, f=0.3) -> (s? t:f=w366:dbl)
            }
          }
          "f" <- w334
        }
        frame #2 {
          n262 = local read "Rright"() -> (w369:dbl)
          n263 = local read "Rleft"() -> (w370:dbl)
          n264 = disable-structure shown="Enabled" {
            disable-tunnel: w369 -> [w381 w388 _]
            disable-tunnel: w370 -> [w380 w389 _]
            disable-tunnel: [w377 w384 TRUE] -> w371
            frame Disabled {
              n265 = Sign(1:w381) -> (0:w379:dbl)
              n266 = Sign(1:w380) -> (0:w378:dbl)
              n267 = Equal?(x=w379, y=w378) -> (x = y?=w377:bool)
            }
            frame Enabled {
              w386 = inf
              n268 = Absolute Value(x=w388) -> (abs(x)=w387:dbl)
              n269 = Absolute Value(x=w389) -> (abs(x)=w385:dbl)
              n270 = Not Equal?(x=w387, y=w386) -> (x != y?=w383:bool)
              n271 = Not Equal?(x=w386, y=w385) -> (x != y?=w382:bool)
              n272 = Or(x=w383, y=w382) -> (x .or. y?=w384:bool)
            }
            frame Disabled {
            }
          }
          n273 = case shown="False" w371 {
            tunnel: w369 -> [_ w427]
            tunnel: w370 -> [_ w426]
            tunnel: [0.5 w425] -> w372
            frame False {
              n274 = local read "Coeff right"() -> (w395:dbl[])
              n275 = local read "Coeff left"() -> (w396:dbl[])
              n276 = Empty Array?(array=w395) -> (empty?=w394:bool)
              n277 = Empty Array?(array=w396) -> (empty?=w392:bool)
              n278 = Exclusive Or(1:w394, 2:w392) -> (0:w393:bool)
              n279 = case shown="False" w393 {
                tunnel: w392 -> [w397 w406]
                frame False {
                  n280 = case shown="True" w397 {
                    frame False {
                      w399 = 0.5
                      n281 = local read "Coeff right"() -> (w402:dbl[])
                      n282 = local read "Coeff left"() -> (w404:dbl[])
                      n283 = Decrement(x=w399) -> (x-1=w403:dbl)
                      n284 = Multiply(x=w404, y=w399) -> (x*y=w401:dbl[])
                      n285 = Multiply(x=w403, y=w402) -> (x*y=w400:dbl[])
                      n286 = Subtract(x=w401, y=w400) -> (x-y=w398:dbl[])
                      n287 = global write "G_SEN.vi" "Lane_C_M"(w398) -> ()
                    }
                    frame True {
                      n288 = local read "Coeff left"() -> (w405:dbl[])
                      n289 = global write "G_SEN.vi" "Lane_C_M"(w405) -> ()
                    }
                  }
                }
                frame True {
                  n290 = case shown="False" w406 {
                    frame False {
                      n291 = global read "G_SEN.vi" "vision lane width"() -> (w410:dbl)
                      n292 = local read "Coeff left"() -> (w415:dbl[])
                      n293 = Index Array(array=w415, index=0) -> (element=w413:dbl)
                      n294 = Multiply(x=w410, y=0.5) -> (x*y=w408:dbl)
                      n295 = Add(x=w413, y=w408) -> (x+y=w412:dbl)
                      n296 = Replace Array Subset(array=w415, new element=w412, index=0) -> (w407:dbl[])
                      n297 = global write "G_SEN.vi" "Lane_C_M"(w407) -> ()
                    }
                    frame True {
                      n298 = global read "G_SEN.vi" "vision lane width"() -> (w419:dbl)
                      n299 = local read "Coeff right"() -> (w424:dbl[])
                      n300 = Index Array(array=w424, index=0) -> (element=w422:dbl)
                      n301 = Multiply(x=w419, y=0.5) -> (x*y=w417:dbl)
                      n302 = Subtract(x=w422, y=w417) -> (x-y=w421:dbl)
                      n303 = Replace Array Subset(array=w424, new element=w421, index=0) -> (w416:dbl[])
                      n304 = global write "G_SEN.vi" "Lane_C_M"(w416) -> ()
                    }
                  }
                }
              }
            }
            frame True {
              n305 = disable-structure shown="Enabled" {
                disable-tunnel: w427 -> [w436 w660]
                disable-tunnel: w426 -> [w435 w659]
                disable-tunnel: [_ w588] -> w425
                frame Disabled {
                  n306 = Absolute Value(x=w436) -> (abs(x)=w458:dbl)
                  n307 = Absolute Value(x=w435) -> (abs(x)=w457:dbl)
                  n308 = global read "G_ALL.vi" "CARSPEC"() -> (w453:T4)
                  n309 = global read "G_ALL.vi" "CARSPEC"() -> (w474:T4)
                  n310 = Build Array(w458, w457) -> (w456:dbl[])
                  n311 = Unbundle By Name(w453) -> ("af"=w452:dbl, "Overall width"=w442:dbl)
                  n312 = Unbundle By Name(w474) -> ("Overall width"=w463:dbl, "af"=w471:dbl, "Overall width"=w459:dbl)
                  n313 = Array Max & Min(array=w456) -> (min value=w449:dbl, min index (indices)=w455:i32)  [unwired: 2 out]
                  n314 = Add(x=w449, y=w463) -> (x+y=w473:dbl)
                  n315 = Square(x=w449) -> (x^2=w440:dbl)
                  n316 = Square(x=w452) -> (x^2=w439:dbl)
                  n317 = Multiply(x=w442, y=0.5) -> (x*y=w441:dbl)
                  n318 = Square(x=w473) -> (x^2=w472:dbl)
                  n319 = Square(x=w471) -> (x^2=w464:dbl)
                  n320 = Subtract(x=w440, y=w439) -> (x-y=w434:dbl)
                  n321 = Multiply(x=w459, y=0.5) -> (x*y=w460:dbl)
                  n322 = Add(x=w472, y=w464) -> (x+y=w470:dbl)
                  n323 = Square Root(x=w434) -> (sqrt(x)=w451:dbl)
                  n324 = global read "G_SEN.vi" "vision lane width"() -> (w445:dbl)
                  n325 = global read "G_SEN.vi" "vision lane width"() -> (w469:dbl)
                  n326 = Subtract(x=w451, y=w442) -> (x-y=w450:dbl)
                  n327 = Square Root(x=w470) -> (sqrt(x)=w468:dbl)
                  n328 = Subtract(x=w449, y=w450) -> (x-y=w444:dbl)
                  n329 = Subtract(x=w468, y=w449) -> (x-y=w467:dbl)
                  n330 = Subtract(x=w445, y=w444) -> (x-y=w446:dbl)
                  n331 = Subtract(x=w469, y=w467) -> (x-y=w466:dbl)
                  n332 = global read "G_SEN.vi" "vision lane width"() -> (w430:dbl)
                  n333 = global read "G_SEN.vi" "vision lane width"() -> (w437:dbl)
                  n334 = Multiply(x=w446, y=0.5) -> (x*y=w448:dbl)
                  n335 = Multiply(x=w466, y=0.5) -> (x*y=w461:dbl)
                  n336 = Compound Arithmetic op=ADD(w448, w441) -> (w438:dbl)
                  n337 = Compound Arithmetic op=ADD(w461, w460) -> (w454:dbl)
                  n338 = Subtract(x=w437, y=w438) -> (x-y=w432:dbl)
                  n339 = Less Than 0?(x=w434) -> (x < 0?=w433:bool)
                  n340 = Multiply(x=0.5 ("y"), y=w430) -> (x*y=w429:dbl)
                  n341 = Select(t=w429, s=w433, f=w432) -> (s? t:f=w431:dbl)
                  n342 = case shown="1" w455 {
                    tunnel: w454 -> [w476 w524]
                    tunnel: w431 -> [w475 w522]
                    frame 0, Default {
                      n343 = local read "Rright"() -> (w478:dbl)
                      n344 = Greater Than 0?(x=w478) -> (x > 0?=w477:bool)
                      n345 = case shown="True" w477 {
                        tunnel: w476 -> [_ w499]
                        tunnel: w475 -> [w481 w498]
                        frame False {
                          n346 = local read "Coeff left"() -> (w480:dbl[])
                          n347 = Empty Array?(array=w480) -> (empty?=w479:bool)
                          n348 = case shown="True" w479 {
                            tunnel: w481 -> [w482 w491]
                            frame False {
                              n349 = global read "G_SEN.vi" "vision lane width"() -> (w490:dbl)
                              n350 = Divide(x=w482, y=w490) -> (x/y=w488:dbl)
                              n351 = local read "Coeff right"() -> (w486:dbl[])
                              n352 = local read "Coeff left"() -> (w489:dbl[])
                              n353 = Decrement(x=w488) -> (x-1=w487:dbl)
                              n354 = Multiply(x=w489, y=w488) -> (x*y=w485:dbl[])
                              n355 = Multiply(x=w487, y=w486) -> (x*y=w484:dbl[])
                              n356 = Subtract(x=w485, y=w484) -> (x-y=w483:dbl[])
                              n357 = global write "G_SEN.vi" "Lane_C_M"(w483) -> ()
                            }
                            frame True {
                              n358 = local read "Coeff right"() -> (w497:dbl[])
                              n359 = Index Array(array=w497, index=0) -> (element=w495:dbl)
                              n360 = Subtract(x=w495, y=w491) -> (x-y=w494:dbl)
                              n361 = Replace Array Subset(array=w497, new element=w494, index=0) -> (w492:dbl[])
                              n362 = global write "G_SEN.vi" "Lane_C_M"(w492) -> ()
                            }
                          }
                        }
                        frame True {
                          n363 = local read "Coeff left"() -> (w501:dbl[])
                          n364 = Empty Array?(array=w501) -> (empty?=w500:bool)
                          n365 = case shown="True" w500 {
                            tunnel: w499 -> [w505 w515]
                            tunnel: w498 -> [w506 _]
                            frame False {
                              n366 = Add(x=w506, y=w505) -> (x+y=w504:dbl)
                              n367 = global read "G_SEN.vi" "vision lane width"() -> (w514:dbl)
                              n368 = Multiply(x=w504, y=0.5) -> (x*y=w502:dbl)
                              n369 = Divide(x=w502, y=w514) -> (x/y=w512:dbl)
                              n370 = local read "Coeff right"() -> (w510:dbl[])
                              n371 = local read "Coeff left"() -> (w513:dbl[])
                              n372 = Decrement(x=w512) -> (x-1=w511:dbl)
                              n373 = Multiply(x=w513, y=w512) -> (x*y=w509:dbl[])
                              n374 = Multiply(x=w511, y=w510) -> (x*y=w508:dbl[])
                              n375 = Subtract(x=w509, y=w508) -> (x-y=w507:dbl[])
                              n376 = global write "G_SEN.vi" "Lane_C_M"(w507) -> ()
                            }
                            frame True {
                              n377 = local read "Coeff right"() -> (w521:dbl[])
                              n378 = Index Array(array=w521, index=0) -> (element=w519:dbl)
                              n379 = Subtract(x=w519, y=w515) -> (x-y=w518:dbl)
                              n380 = Replace Array Subset(array=w521, new element=w518, index=0) -> (w516:dbl[])
                              n381 = global write "G_SEN.vi" "Lane_C_M"(w516) -> ()
                            }
                          }
                        }
                      }
                    }
                    frame 1 {
                      n382 = local read "Rleft"() -> (w525:dbl)
                      n383 = Less Than 0?(x=w525) -> (x < 0?=w523:bool)
                      n384 = case shown="False" w523 {
                        tunnel: w524 -> [_ w546]
                        tunnel: w522 -> [w528 w545]
                        frame False {
                          n385 = local read "Coeff right"() -> (w527:dbl[])
                          n386 = Empty Array?(array=w527) -> (empty?=w526:bool)
                          n387 = case shown="False" w526 {
                            tunnel: w528 -> [w529 w538]
                            frame False {
                              n388 = global read "G_SEN.vi" "vision lane width"() -> (w537:dbl)
                              n389 = Divide(x=w529, y=w537) -> (x/y=w535:dbl)
                              n390 = local read "Coeff right"() -> (w536:dbl[])
                              n391 = local read "Coeff left"() -> (w533:dbl[])
                              n392 = Decrement(x=w535) -> (x-1=w534:dbl)
                              n393 = Multiply(x=w536, y=w535) -> (x*y=w532:dbl[])
                              n394 = Multiply(x=w534, y=w533) -> (x*y=w531:dbl[])
                              n395 = Subtract(x=w532, y=w531) -> (x-y=w530:dbl[])
                              n396 = global write "G_SEN.vi" "Lane_C_M"(w530) -> ()
                            }
                            frame True {
                              n397 = local read "Coeff left"() -> (w544:dbl[])
                              n398 = Index Array(array=w544, index=0) -> (element=w542:dbl)
                              n399 = Add(x=w542, y=w538) -> (x+y=w541:dbl)
                              n400 = Replace Array Subset(array=w544, new element=w541, index=0) -> (w539:dbl[])
                              n401 = global write "G_SEN.vi" "Lane_C_M"(w539) -> ()
                            }
                          }
                        }
                        frame True {
                          n402 = local read "Coeff right"() -> (w548:dbl[])
                          n403 = Empty Array?(array=w548) -> (empty?=w547:bool)
                          n404 = case shown="False" w547 {
                            tunnel: w546 -> [w550 w562]
                            tunnel: w545 -> [w551 _]
                            frame False {
                              n405 = Add(x=w551, y=w550) -> (x+y=w553:dbl)
                              n406 = global read "G_SEN.vi" "vision lane width"() -> (w561:dbl)
                              n407 = Multiply(x=w553, y=0.5) -> (x*y=w549:dbl)
                              n408 = Divide(x=w549, y=w561) -> (x/y=w559:dbl)
                              n409 = local read "Coeff right"() -> (w560:dbl[])
                              n410 = local read "Coeff left"() -> (w557:dbl[])
                              n411 = Decrement(x=w559) -> (x-1=w558:dbl)
                              n412 = Multiply(x=w560, y=w559) -> (x*y=w556:dbl[])
                              n413 = Multiply(x=w558, y=w557) -> (x*y=w555:dbl[])
                              n414 = Subtract(x=w556, y=w555) -> (x-y=w554:dbl[])
                              n415 = global write "G_SEN.vi" "Lane_C_M"(w554) -> ()
                            }
                            frame True {
                              n416 = local read "Coeff left"() -> (w568:dbl[])
                              n417 = Index Array(array=w568, index=0) -> (element=w566:dbl)
                              n418 = Add(x=w566, y=w562) -> (x+y=w565:dbl)
                              n419 = Replace Array Subset(array=w568, new element=w565, index=0) -> (w563:dbl[])
                              n420 = global write "G_SEN.vi" "Lane_C_M"(w563) -> ()
                            }
                          }
                        }
                      }
                    }
                  }
                }
                frame Enabled {
                  n421 = Build Array(w660, w659) -> (w634:dbl[])
                  n422 = global read "G_ALL.vi" "CARSPEC"() -> (w657:T4)
                  n423 = Absolute Value(x=w634) -> (abs(x)=w658:dbl[])
                  n424 = Unbundle By Name(w657) -> ("Overall width"=w656:dbl, "af"=w654:dbl, "Overall width"=w583:dbl)
                  n425 = Array Max & Min(array=w658) -> (max value=w636:dbl, min value=w593:dbl, min index (indices)=w633:i32)  [unwired: 1 out]
                  n426 = global read "G_ALL.vi" "CARSPEC"() -> (w645:T4)
                  n427 = Index Array(array=w634, index=w633) -> (element=w632:dbl)
                  n428 = Add(x=w593, y=w656) -> (x+y=w655:dbl)
                  n429 = Square(x=w654) -> (x^2=w652:dbl)
                  n430 = Not Equal?(x=inf, y=w636) -> (x != y?=w631:bool)
                  n431 = Unbundle By Name(w645) -> ("Overall width"=w577:dbl, "af"=w644:dbl)
                  n432 = Select(t=w636, s=w631, f=w593) -> (s? t:f=w635:dbl)
                  n433 = Square(x=w655) -> (x^2=w653:dbl)
                  n434 = Multiply(x=w583, y=0.5) -> (x*y=w582:dbl)
                  n435 = Square(x=w635) -> (x^2=w642:dbl)
                  n436 = Square(x=w644) -> (x^2=w643:dbl)
                  n437 = Add(x=w653, y=w652) -> (x+y=w651:dbl)
                  n438 = global read "G_SEN.vi" "vision lane width"() -> (w648:dbl)
                  n439 = Subtract(x=w642, y=w643) -> (x-y=w594:dbl)
                  n440 = Square Root(x=w651) -> (sqrt(x)=w650:dbl)
                  n441 = Add(x=w582, y=0.1) -> (x+y=w579:dbl)
                  n442 = Subtract(x=w593, y=w650) -> (x-y=w649:dbl)
                  n443 = Max & Min(x=w594, y=w593) -> (max(x,y)=w592:dbl)  [unwired: 1 out]
                  n444 = global read "G_SEN.vi" "vision lane width"() -> (w640:dbl)
                  n445 = Compound Arithmetic op=ADD(w649, w583, w648) -> (w647:dbl)
                  n446 = Square Root(x=w592) -> (sqrt(x)=w641:dbl)
                  n447 = Multiply(x=0.5, y=w577) -> (x*y=w574:dbl)
                  n448 = Subtract(x=w635, y=w641) -> (x-y=w575:dbl)
                  n449 = Multiply(x=w647, y=0.5) -> (x*y=w580:dbl)
                  n450 = Max & Min(x=w580, y=w579) -> (max(x,y)=w578:dbl)  [unwired: 1 out]
                  n451 = Compound Arithmetic op=ADD(w575, w640) -> (w638:dbl)
                  n452 = Compound Arithmetic op=ADD(0.1 ("value"), w574, w575) -> (w571:dbl)
                  n453 = Multiply(x=w638, y=0.5) -> (x*y=w572:dbl)
                  n454 = Max & Min(x=w571, y=w572) -> (max(x,y)=w570:dbl)  [unwired: 1 out]
                  n455 = case shown="True" w631 {
                    tunnel: w633 -> [w665 w683]
                    tunnel: w632 -> [w664 _]
                    tunnel: w578 -> [w663 w686]
                    tunnel: [w662 w678] -> w630
                    tunnel: w570 -> [w661 w688]
                    frame False {
                      n456 = case shown="1" w665 {
                        tunnel: w664 -> [w670 w677]
                        tunnel: w663 -> [w667 w675]
                        tunnel: [w666 w671] -> w662
                        tunnel: w661 -> [w668 w674]
                        frame 0, Default {
                          n457 = Less Than 0?(x=w670) -> (x < 0?=w669:bool)
                          n458 = Select(t=w668, s=w669, f=w667) -> (s? t:f=w666:dbl)
                        }
                        frame 1 {
                          n459 = Greater Than 0?(x=w677) -> (x > 0?=w676:bool)
                          n460 = Select(t=w674, s=w676, f=w675) -> (s? t:f=w672:dbl)
                          n461 = global read "G_SEN.vi" "vision lane width"() -> (w673:dbl)
                          n462 = Subtract(x=w673, y=w672) -> (x-y=w671:dbl)
                        }
                      }
                    }
                    frame True {
                      n463 = Equal To 0?(x=w683) -> (x = 0?=w682:bool)
                      n464 = global read "G_SEN.vi" "vision lane width"() -> (w689:dbl)
                      n465 = Subtract(x=w689, y=w688) -> (x-y=w687:dbl)
                      n466 = Add(x=w687, y=w686) -> (x+y=w684:dbl)
                      n467 = global read "G_SEN.vi" "vision lane width"() -> (w681:dbl)
                      n468 = Multiply(x=w684, y=0.5) -> (x*y=w680:dbl)
                      n469 = Subtract(x=w681, y=w680) -> (x-y=w679:dbl)
                      n470 = Select(t=w680, s=w682, f=w679) -> (s? t:f=w678:dbl)
                    }
                  }
                  n471 = global read "G_SEN.vi" "vision lane width"() -> (w629:dbl)
                  n472 = local read "Coeff right"() -> (w569:dbl[])
                  n473 = local read "Coeff left"() -> (w603:dbl[])
                  n474 = global read "G_SEN.vi" "vision lane width"() -> (w614:dbl)
                  n475 = global read "G_SEN.vi" "vision lane width"() -> (w605:dbl)
                  n476 = Divide(x=w630, y=w629) -> (x/y=w590:dbl)
                  n477 = local read "poly"() -> (w620:i32)
                  n478 = local read "poly"() -> (w599:i32)
                  n479 = Increment(x=w620) -> (x+1=w619:i32)
                  n480 = Increment(x=w599) -> (x+1=w600:i32)
                  n481 = Index Array(array=w569, index #1=0 ("index")) -> (element #1=w615:dbl, element #2=w596:dbl)  [unwired: 1 in]
                  n482 = Index Array(array=w603, index #1=0 ("index")) -> (element #1=w604:dbl, element #2=w595:dbl)  [unwired: 1 in]
                  n483 = Subtract(x=0.5, y=w590) -> (x-y=w587:dbl)
                  n484 = local read "Coeff right"() -> (w609:dbl[])
                  n485 = Subtract(x=w615, y=w614) -> (x-y=w613:dbl)
                  n486 = Add(x=w604, y=w605) -> (x+y=w606:dbl)
                  n487 = Initialize Array(0.0 ("element"), w619) -> (w618:dbl[])
                  n488 = Initialize Array(0.0 ("element"), w600) -> (w601:dbl[])
                  n489 = local read "Coeff left"() -> (w623:dbl[])
                  n490 = Multiply(x=w587, y="lane_gain") -> (x*y=w586:dbl)
                  n491 = Empty Array?(array=w609) -> (empty?=w611:bool)
                  n492 = Empty Array?(array=w623) -> (empty?=w624:bool)
                  n493 = Replace Array Subset(array=w618, new element #1=w613, index #1=0 ("index"), new element #2=w596) -> (w617:dbl[])  [unwired: 1 in]
                  n494 = Replace Array Subset(array=w601, new element #1=w606, index #1=0 ("index"), new element #2=w595) -> (w597:dbl[])  [unwired: 1 in]
                  n495 = Not(x=w611) -> (.not. x?=w610:bool)
                  n496 = Subtract(x=0.5 ("y"), y=w586) -> (x-y=w588:dbl)
                  n497 = Select(t=w617, s=w624, f=w623) -> (s? t:f=w622:dbl[])
                  n498 = Select(t=w609, s=w610, f=w597) -> (s? t:f=w608:dbl[])
                  n499 = Decrement(x=w588) -> (x-1=w628:dbl)
                  n500 = Multiply(x=w622, y=w588) -> (x*y=w626:dbl[])
                  n501 = Multiply(x=w628, y=w608) -> (x*y=w627:dbl[])
                  n502 = Subtract(x=w626, y=w627) -> (x-y=w625:dbl[])
                  n503 = global write "G_SEN.vi" "Lane_C_M"(w625) -> ()
                }
              }
            }
          }
          n504 = Subtract(x=0.5, y=w372) -> (x-y=w374:dbl)
          n505 = Multiply(x=w374, y=2.0) -> (x*y=→"ratio(-1:left1:right)":dbl)
        }
        frame #3 {
          n506 = global read "G_SEN.vi" "Lane_C_M"() -> (w719:dbl[])
          n507 = Array Size(array=w719) -> (size(s)=w710:i32)
          n508 = global read "G_ALL.vi" "map_track 2"() -> (w708:dbl[][])
          n509 = Decrement(x=w710) -> (x-1=w723:i32)
          n510 = Initialize Array(0.0 ("element"), w723) -> (w721:dbl[])
          n511 = local read "Coeff stop"() -> (w716:dbl[])
          n512 = local read "f"() -> (w720:dbl)
          n513 = Array Subset(array=w708, index (row)=30 ("index"), length (row)=10 ("length")) -> (w705:dbl[][])  [unwired: 2 in]
          n514 = Insert Into Array(array=w721, index=0, new element=w720) -> (w717:dbl[])
          n515 = Index Array(array=w716, index=0) -> (element=w703:dbl)
          n516 = Index Array(array=w705, index (col)=1 ("disabled index (col)")) -> (element=w691:dbl[])  [unwired: 1 in]
          n517 = Subtract(x=w703, y=2.0) -> (x-y=w690:dbl)
          n518 = Add(x=w719, y=w717) -> (x+y=w713:dbl[])
          n519 = Less?(x=w703, y=7.0) -> (x < y?=w697:bool)
          n520 = Initialize Array(0.0 ("element"), w710) -> (w709:dbl[])
          n521 = Greater?(x=w691, y=w690) -> (0:w701:bool[])
          n522 = Boolean To (0,1)(Boolean=w701) -> (0, 1=w700:i16[])
          n523 = Add Array Elements(numeric array=w700) -> (sum=w699:i16)
          n524 = Select(t=w709, s=w697, f=w713) -> (s? t:f=w712:dbl[])
          n525 = global write "G_SEN.vi" "Lane_C_M"(w712) -> ()
          n526 = Greater?(x=w699, y=i16 0) -> (0:w696:bool)
          n527 = And(x=w697, y=w696) -> (x .and. y?=w695:bool)
          n528 = Select(t=-0.1, s=w695, f=0.0) -> (s? t:f=→"stop_shift":dbl)
        }
        frame #4 {
          n529 = global read "G_SEN.vi" "Lane_C_M"() -> (w724:dbl[])
          "Lane_C_M" <- w724
          n530 = Index Array(array=w724, index=0) -> (element=w726:dbl)
          n531 = Not A Number/Path/Refnum?(number/path/refnum=w726) -> (NaN/Path/Refnum?=w727:bool)
          n532 = case shown="True" w727 {
            selector: w727 -> [_ w728]
            frame False {
            }
            frame True {
              "NaN/Path/Refnum?" <- w728
            }
          }
        }
      }
    }
    frame #3 {
      n533 = global read "G_ALL.vi" "map_track 2"() -> (w732:dbl[][])
      n534 = Empty Array?(array=w732) -> (empty?=w730:bool)
      n535 = case shown="False" w730 {
        tunnel: [w737 _] -> w729
        tunnel: [w736 _] -> w733
        tunnel: [w735 _] -> w731
        tunnel: w732 -> [w734 _]
        frame False {
          n536 = flat-sequence {
            tunnel: w734 -> [w738]
            tunnel: [w860] -> w737
            tunnel: [w859] -> w736
            tunnel: [w858] -> w735
            frame #0 {
              n537 = global read "G_ALL.vi" "dist"() -> (w743:dbl[])
              n538 = Threshold 1D Array(2:-4.0 ("threshold y"), 3:w743) -> (0:w741:dbl)  [unwired: 1 in]
              n539 = Round Toward +Infinity(x=w741) -> (ceil(x): smallest int >= x=w739:dbl)
              n540 = Array Subset(array=w738, index (row)=w739) -> (→"map_track":dbl[][])  [unwired: 3 in]
            }
            frame #1 {
              n541 = local read "d_safe"() -> (w750:dbl)
              n542 = local read "y 2"() -> (w747:dbl[])
              n543 = local read "map_track"() -> (w744:dbl[][])
              n544 = Array Size(array=w747) -> (size(s)=w746:i32)
              n545 = local read "x 2"() -> (w751:dbl[])
              n546 = Subtract(x=w750, y=0.2) -> (x-y=w749:dbl)
              n547 = for {
                N: w746 -> [_]
                tunnel: w747 -> [w758] mode=indexing
                tunnel: w751 -> [w759] mode=indexing
                tunnel: w744 -> [w764]
                tunnel: w749 -> [w760]
                tunnel: [w756] -> w752 mode=indexing
                tunnel: [w753] -> w745 mode=indexing
                i -> [w754]
                n548 = Build Array(w759, w758) -> (w757:dbl[])
                n549 = Index Array(array=w764, index (col) #1=0 ("disabled index (col)")) -> (element #1=w772:dbl[], element #2=w771:dbl[])  [unwired: 3 in]
                n550 = Subtract(x=w759, y=w772) -> (x-y=w769:dbl[])
                n551 = Subtract(x=w771, y=w758) -> (x-y=w770:dbl[])
                n552 = Square(x=w769) -> (x^2=w768:dbl[])
                n553 = Square(x=w770) -> (x^2=w767:dbl[])
                n554 = Add(x=w768, y=w767) -> (x+y=w766:dbl[])
                n555 = Square Root(x=w766) -> (sqrt(x)=w765:dbl[])
                n556 = Array Max & Min(array=w765) -> (min value=w761:dbl, min index (indices)=w763:i32)  [unwired: 2 out]
                n557 = Less Or Equal?(x=w760, y=w761) -> (x <= y?=w762:bool)
                n558 = case shown="True" w762 {
                  tunnel: w764 -> [_ w795]
                  tunnel: w763 -> [_ w794]
                  tunnel: w757 -> [_ w788]
                  tunnel: [_ w776] -> w756
                  frame False {
                  }
                  frame True {
                    n559 = Decrement(x=w794) -> (x-1=w793:i32)
                    n560 = Max & Min(x=w793, y=0) -> (max(x,y)=w792:i32)  [unwired: 1 out]
                    n561 = Index Array(array=w795, index (row) #1=w792) -> (element #1=w789:dbl[], element #2=w790:dbl[])  [unwired: 3 in]
                    n562 = Subtract(x=w788, y=w789) -> (x-y=w785:dbl[])
                    n563 = Subtract(x=w790, y=w789) -> (x-y=w787:dbl[])
                    n564 = Index Array(array=w785, index #1=0 ("index"), index #2=1 ("index")) -> (element #1=w779:dbl, element #2=w781:dbl)
                    n565 = Index Array(array=w787, index #1=0 ("index"), index #2=1 ("index")) -> (element #1=w780:dbl, element #2=w778:dbl)
                    n566 = Multiply(x=w779, y=w778) -> (x*y=w775:dbl)
                    n567 = Multiply(x=w781, y=w780) -> (x*y=w774:dbl)
                    n568 = Subtract(x=w775, y=w774) -> (x-y=w777:dbl)
                    n569 = Sign(1:w777) -> (0:w776:dbl)
                  }
                }
                n570 = local read "w"() -> (w755:dbl[])
                n571 = Index Array(array=w755, index=w754) -> (element=w753:dbl)
              }
              "w 2" <- w752
              n572 = local write "w"(w745) -> ()
            }
            frame #2 {
              n573 = local read "w 2"() -> (w813:dbl[])
              n574 = local read "w 2"() -> (w814:dbl[])
              n575 = local read "w"() -> (w816:dbl[])
              n576 = local read "w"() -> (w806:dbl[])
              n577 = local read "w"() -> (w819:dbl[])
              n578 = local read "w"() -> (w803:dbl[])
              n579 = Greater Or Equal?(x=w813, y=1.0) -> (x >= y?=w808:bool[])
              n580 = Greater Or Equal?(x=w816, y=1.0) -> (x >= y?=w810:bool[])
              n581 = Less Or Equal?(x=w806, y=-1.0) -> (x <= y?=w805:bool[])
              n582 = Less Or Equal?(x=w819, y=-1.0) -> (x <= y?=w811:bool[])
              n583 = Less Or Equal?(x=w814, y=-1.0) -> (x <= y?=w809:bool[])
              n584 = Greater Or Equal?(x=w803, y=1.0) -> (x >= y?=w801:bool[])
              n585 = Or(x=w810, y=w808) -> (x .or. y?=w798:bool[])
              n586 = Not(x=w805) -> (.not. x?=w804:bool[])
              n587 = Or(x=w811, y=w809) -> (x .or. y?=w799:bool[])
              n588 = Not(x=w801) -> (.not. x?=w800:bool[])
              n589 = local read "x 2"() -> (w820:dbl[])
              n590 = local read "y 2"() -> (w821:dbl[])
              n591 = local read "x 2"() -> (w843:dbl[])
              n592 = local read "y 2"() -> (w842:dbl[])
              n593 = And(x=w798, y=w804) -> (x .and. y?=w796:bool[])
              n594 = And(x=w799, y=w800) -> (x .and. y?=w797:bool[])
              n595 = Boolean To (0,1)(Boolean=w796) -> (0, 1=w826:i16[])
              n596 = Boolean To (0,1)(Boolean=w797) -> (0, 1=w837:i16[])
              n597 = Build Cluster Array(w796, w820, w821) -> (w822:cluster{bool, dbl, dbl}[])
              n598 = Build Cluster Array(w797, w843, w842) -> (w841:cluster{bool, dbl, dbl}[])
              n599 = To Long Integer(number=w826) -> (32bit integer=w827:i32[])
              n600 = To Long Integer(number=w837) -> (32bit integer=w836:i32[])
              n601 = Sort 1D Array(array=w822) -> (sorted array=w823:cluster{bool, dbl, dbl}[])
              n602 = Sort 1D Array(array=w841) -> (sorted array=w840:cluster{bool, dbl, dbl}[])
              n603 = Add Array Elements(numeric array=w827) -> (sum=w825:i32)
              n604 = Add Array Elements(numeric array=w836) -> (sum=w838:i32)
              n605 = Reverse 1D Array(array=w823) -> (reversed array=w824:cluster{bool, dbl, dbl}[])
              n606 = Reverse 1D Array(array=w840) -> (reversed array=w839:cluster{bool, dbl, dbl}[])
              n607 = for {
                N: w825 -> [_]
                tunnel: w824 -> [w847] mode=indexing
                tunnel: [w846] -> w829 mode=indexing
                tunnel: [w845] -> w828 mode=indexing
                tunnel: [w844] -> _
                i -> [w844]
                n608 = Unbundle(w847) -> (w846:dbl, w845:dbl)  [unwired: 1 out]
              }
              n609 = for {
                N: w838 -> [_]
                tunnel: w839 -> [w851] mode=indexing
                tunnel: [w850] -> w834 mode=indexing
                tunnel: [w849] -> w835 mode=indexing
                tunnel: [w848] -> _
                i -> [w848]
                n610 = Unbundle(w851) -> (w850:dbl, w849:dbl)  [unwired: 1 out]
              }
              n611 = Build Array(w829, w828) -> (w830:dbl[][])
              n612 = Build Array(w834, w835) -> (w833:dbl[][])
              n613 = Transpose 2D Array(2D array=w830) -> (transposed array=→"lane_right_pt":dbl[][])
              n614 = Transpose 2D Array(2D array=w833) -> (transposed array=→"lane_left_pt":dbl[][])
            }
            frame #3 {
              n615 = local read "lane_right_pt"() -> (w883:dbl[][])
              n616 = local read "lane_left_pt"() -> (w881:dbl[][])
              n617 = Empty Array?(array=w883) -> (empty?=w882:bool)
              n618 = Empty Array?(array=w881) -> (empty?=w880:bool)
              n619 = case shown="False" w882 {
                tunnel: [w936 _] -> w877
                tunnel: [w935 _] -> w874
                frame False {
                  n620 = local read "map_track"() -> (w934:dbl[][])
                  n621 = local read "lane_right_pt"() -> (w938:dbl[][])
                  n622 = local read "map_track"() -> (w942:dbl[][])
                  n623 = Index Array(array=w934, index (col)=1 ("disabled index (col)")) -> ()  [unwired: 1 in, 1 out]
                  n624 = Index Array(array=w938, index (col) #1=0 ("disabled index (col)")) -> (element #1=w940:dbl[], element #2=w941:dbl[])  [unwired: 3 in]
                  n625 = Delete From Array(array=w942, index (row)=0) -> (deleted portion=w945:dbl[], array with subset deleted=w943:dbl[][])  [unwired: 2 in]
                  n626 = local read "d_safe"() -> (w937:dbl)
                  n627 = for {
                    tunnel: w940 -> [w977]
                    tunnel: w941 -> [w976]
                    tunnel: w943 -> [w967] mode=indexing
                    shift-right: [w967] -> _
                    shift-left: w945 -> [w966]
                    tunnel: [w955] -> w946 mode=indexing
                    tunnel: [w953] -> w947 mode=indexing
                    tunnel: w937 -> [w954]
                    n628 = Subtract(x=w967, y=w966) -> (x-y=w965:dbl[])
                    n629 = Index Array(array=w967) -> (element #1=w969:dbl, element #2=w968:dbl)  [unwired: 2 in]
                    n630 = Subtract(x=w977, y=w969) -> (x-y=w975:dbl[])
                    n631 = Subtract(x=w976, y=w968) -> (x-y=w974:dbl[])
                    n632 = Index Array(array=w965, index #1=1 ("index"), index #2=0 ("index")) -> (element #1=w962:dbl, element #2=w961:dbl)
                    n633 = Square(x=w975) -> (x^2=w972:dbl[])
                    n634 = Square(x=w974) -> (x^2=w973:dbl[])
                    n635 = Inverse Tangent (2 Input)(1:w961, 2:w962) -> (0:w960:dbl)
                    n636 = Add(x=w972, y=w973) -> (x+y=w971:dbl[])
                    n637 = call "headingoperater.vi"("h1"=1.5707963267948966, "h2"=w960) -> ("h2+h1"=w953:dbl)  [unwired: 8 in, 1 out]
                    n638 = Square Root(x=w971) -> (sqrt(x)=w970:dbl[])
                    n639 = Array Max & Min(array=w970) -> (min value=w958:dbl)  [unwired: 3 out]
                    n640 = Subtract(x=w954, y=w958) -> (x-y=w957:dbl)
                    n641 = Max & Min(x=w957, y=0.0) -> (max(x,y)=w955:dbl)  [unwired: 1 out]
                  }
                  n642 = Polar To Re/Im(2:w947, 3:w946) -> (0:w949:dbl[], 1:w948:dbl[])
                  n643 = Add Array Elements(numeric array=w948) -> (sum=w951:dbl)
                  n644 = Add Array Elements(numeric array=w949) -> (sum=w950:dbl)
                  n645 = Array Size(array=w949) -> (size(s)=w952:i32)
                  n646 = Divide(x=w951, y=w952) -> (x/y=w936:dbl)
                  n647 = Divide(x=w950, y=w952) -> (x/y=w935:dbl)
                }
                frame True {
                }
              }
              n648 = case shown="False" w880 {
                tunnel: [w891 _] -> w868
                tunnel: [w890 _] -> w871
                frame False {
                  n649 = local read "lane_left_pt"() -> (w907:dbl[][])
                  n650 = local read "map_track"() -> (w903:dbl[][])
                  n651 = Index Array(array=w907, index (col) #1=0 ("disabled index (col)")) -> (element #1=w905:dbl[], element #2=w904:dbl[])  [unwired: 3 in]
                  n652 = Delete From Array(array=w903, index (row)=0) -> (deleted portion=w900:dbl[], array with subset deleted=w902:dbl[][])  [unwired: 2 in]
                  n653 = local read "d_safe"() -> (w892:dbl)
                  n654 = for {
                    tunnel: w905 -> [w932]
                    tunnel: w904 -> [w931]
                    tunnel: w902 -> [w922] mode=indexing
                    shift-right: [w922] -> _
                    shift-left: w900 -> [w921]
                    tunnel: [w909] -> w899 mode=indexing
                    tunnel: [w910] -> w898 mode=indexing
                    tunnel: w892 -> [w908]
                    n655 = Subtract(x=w922, y=w921) -> (x-y=w920:dbl[])
                    n656 = Index Array(array=w922) -> (element #1=w924:dbl, element #2=w923:dbl)  [unwired: 2 in]
                    n657 = Subtract(x=w932, y=w924) -> (x-y=w930:dbl[])
                    n658 = Subtract(x=w931, y=w923) -> (x-y=w929:dbl[])
                    n659 = Index Array(array=w920, index #1=1 ("index"), index #2=0 ("index")) -> (element #1=w917:dbl, element #2=w916:dbl)
                    n660 = Square(x=w930) -> (x^2=w927:dbl[])
                    n661 = Square(x=w929) -> (x^2=w928:dbl[])
                    n662 = Inverse Tangent (2 Input)(1:w916, 2:w917) -> (0:w915:dbl)
                    n663 = Add(x=w927, y=w928) -> (x+y=w926:dbl[])
                    n664 = call "headingoperater.vi"("h1"=1.5707963267948966, "h2"=w915) -> ("h2-h1"=w910:dbl)  [unwired: 8 in, 1 out]
                    n665 = Square Root(x=w926) -> (sqrt(x)=w925:dbl[])
                    n666 = Array Max & Min(array=w925) -> (min value=w913:dbl)  [unwired: 3 out]
                    n667 = Subtract(x=w908, y=w913) -> (x-y=w912:dbl)
                    n668 = Max & Min(x=w912, y=0.0) -> (max(x,y)=w909:dbl)  [unwired: 1 out]
                  }
                  n669 = Polar To Re/Im(2:w898, 3:w899) -> (0:w896:dbl[], 1:w897:dbl[])
                  n670 = Add Array Elements(numeric array=w897) -> (sum=w894:dbl)
                  n671 = Add Array Elements(numeric array=w896) -> (sum=w895:dbl)
                  n672 = Array Size(array=w896) -> (size(s)=w893:i32)
                  n673 = Divide(x=w894, y=w893) -> (x/y=w891:dbl)
                  n674 = Divide(x=w895, y=w893) -> (x/y=w890:dbl)
                }
                frame True {
                }
              }
              n675 = Not A Number/Path/Refnum?(number/path/refnum=w877) -> (NaN/Path/Refnum?=w879:bool)
              n676 = Not A Number/Path/Refnum?(number/path/refnum=w874) -> (NaN/Path/Refnum?=w875:bool)
              n677 = Not A Number/Path/Refnum?(number/path/refnum=w868) -> (NaN/Path/Refnum?=w869:bool)
              n678 = Not A Number/Path/Refnum?(number/path/refnum=w871) -> (NaN/Path/Refnum?=w873:bool)
              n679 = local read "map_track"() -> (w889:dbl[][])
              n680 = Select(t=0.0, s=w879, f=w877) -> (s? t:f=w865:dbl)
              n681 = Select(t=0.0, s=w869, f=w868) -> (s? t:f=w864:dbl)
              n682 = Select(t=0.0, s=w875, f=w874) -> (s? t:f=w862:dbl)
              n683 = Select(t=0.0, s=w873, f=w871) -> (s? t:f=w863:dbl)
              n684 = local read "stop_shift"() -> (w855:dbl)
              n685 = Add(x=w865, y=w864) -> (x+y=w866:dbl)
              n686 = Add(x=w862, y=w863) -> (x+y=w854:dbl)
              n687 = Index Array(array=w889, index (col) #1=0 ("disabled index (col)")) -> (element #1=w887:dbl[], element #2=w886:dbl[])  [unwired: 3 in]
              n688 = Not Equal?(x=w855, y=0.0) -> (x != y?=w856:bool)
              n689 = Add(x=w866, y=w887) -> (x+y=w885:dbl[])
              n690 = Multiply(x="x_gain", y=w866) -> (x*y=w860:dbl)
              n691 = Multiply(x=w854, y="y_gain") -> (x*y=w859:dbl)
              n692 = Select(t=w855, s=w856, f=w854) -> (s? t:f=w852:dbl)
              n693 = Add(x=w852, y=w886) -> (x+y=w853:dbl[])
              n694 = Build Array(w885, w853) -> (w884:dbl[][])
              n695 = Transpose 2D Array(2D array=w884) -> (transposed array=w858:dbl[][])
            }
          }
        }
        frame True {
        }
      }
      "map_track 2" <- w731
      "y_shift" <- w733
      "x_shift" <- w729
      n696 = global write "G_SEN.vi" "vision x shift"(w729) -> ()
      n697 = global write "G_SEN.vi" "vision y shift"(w733) -> ()
    }
    frame #4 {
      n698 = disable-structure shown="Enabled" {
        frame Enabled {
          n699 = local read "w 2"() -> (w1016:dbl[])
          n700 = local read "w 2"() -> (w1015:dbl[])
          n701 = local read "w"() -> (→"Waveform Graph":dbl[])
          n702 = local read "w"() -> (w1095:dbl[])
          n703 = local read "w"() -> (w997:dbl[])
          n704 = local read "w"() -> (w1078:dbl[])
          n705 = local read "w"() -> (w1000:dbl[])
          n706 = Greater Or Equal?(x=w1015, y=1.0) -> (x >= y?=w1010:bool[])
          n707 = Less Or Equal?(x=w1095, y=-1.0) -> (x <= y?=w1013:bool[])
          n708 = Less Or Equal?(x=w1016, y=-1.0) -> (x <= y?=w1011:bool[])
          n709 = Greater Or Equal?(x=w997, y=1.0) -> (x >= y?=w995:bool[])
          n710 = Greater Or Equal?(x=w1078, y=1.0) -> (x >= y?=w1012:bool[])
          n711 = Less Or Equal?(x=w1000, y=-1.0) -> (x <= y?=w999:bool[])
          n712 = Or(x=w1013, y=w1011) -> (x .or. y?=w993:bool[])
          n713 = Or(x=w1012, y=w1010) -> (x .or. y?=w991:bool[])
          n714 = Not(x=w995) -> (.not. x?=w994:bool[])
          n715 = Not(x=w999) -> (.not. x?=w998:bool[])
          n716 = And(x=w993, y=w994) -> (x .and. y?=w992:bool[])
          n717 = And(x=w991, y=w998) -> (x .and. y?=w990:bool[])
          n718 = local read "x 2"() -> (w1093:dbl[])
          n719 = local read "y 2"() -> (w1092:dbl[])
          n720 = local read "x 2"() -> (w1080:dbl[])
          n721 = local read "y 2"() -> (w1081:dbl[])
          n722 = Build Cluster Array(w992, w1093, w1092) -> (w1091:cluster{bool, dbl, dbl}[])
          n723 = Build Cluster Array(w990, w1080, w1081) -> (w1082:cluster{bool, dbl, dbl}[])
          n724 = Sort 1D Array(array=w1091) -> (sorted array=w1090:cluster{bool, dbl, dbl}[])
          n725 = Sort 1D Array(array=w1082) -> (sorted array=w1083:cluster{bool, dbl, dbl}[])
          n726 = Reverse 1D Array(array=w1090) -> (reversed array=w1089:cluster{bool, dbl, dbl}[])
          n727 = Reverse 1D Array(array=w1083) -> (reversed array=w1084:cluster{bool, dbl, dbl}[])
          n728 = for {
            tunnel: w1089 -> [w1109] mode=indexing
            tunnel: [w1107] -> w1088 mode=indexing
            tunnel: [w1106] -> w1074 mode=indexing
            tunnel: [w1105] -> w1087
            i -> [w1105]
            stop <- w1108 continue-if-true
            n729 = Unbundle(w1109) -> (w1108:bool, w1107:dbl, w1106:dbl)
          }
          n730 = for {
            tunnel: w1084 -> [w1104] mode=indexing
            tunnel: [w1102] -> w1085 mode=indexing
            tunnel: [w1101] -> w1072 mode=indexing
            tunnel: [w1100] -> w1086
            i -> [w1100]
            stop <- w1103 continue-if-true
            n731 = Unbundle(w1104) -> (w1103:bool, w1102:dbl, w1101:dbl)
          }
          n732 = Array Subset(array=w1088, index=0, length=w1087) -> (w985:dbl[])
          n733 = Array Subset(array=w1085, index=0, length=w1086) -> (w983:dbl[])
          n734 = Array Subset(array=w1074, index=0, length=w1087) -> (w984:dbl[])
          n735 = Array Subset(array=w1072, index=0, length=w1086) -> (w982:dbl[])
          n736 = call "Convert to Dynamic Data4"("Array"=w985) -> ("Dynamic Data Type"=w988:dynamicdata)  [unwired: 3 in]
          n737 = call "Convert to Dynamic Data6"("Array"=w983) -> ("Dynamic Data Type"=w987:dynamicdata)  [unwired: 3 in]
          n738 = Array Max & Min(array=w984) -> (max value=w1009:dbl, min value=w1007:dbl)  [unwired: 2 out]
          n739 = call "Convert to Dynamic Data3"("Array"=w984) -> ("Dynamic Data Type"=w989:dynamicdata)  [unwired: 3 in]
          n740 = Array Max & Min(array=w982) -> (max value=w1005:dbl, min value=w1003:dbl)  [unwired: 2 out]
          n741 = call "Convert to Dynamic Data8"("Array"=w982) -> ("Dynamic Data Type"=w986:dynamicdata)  [unwired: 3 in]
          n742 = Decrement(x=w1009) -> (x-1=w1008:dbl)
          n743 = Increment(x=w1007) -> (x+1=w1006:dbl)
          n744 = Decrement(x=w1005) -> (x-1=w1004:dbl)
          n745 = Increment(x=w1003) -> (x+1=w1002:dbl)
          n746 = local read "map_track"() -> (w1026:dbl[][])
          n747 = Add(x=w1008, y=w1004) -> (x+y=w1045:dbl)
          n748 = Add(x=w1006, y=w1002) -> (x+y=w1041:dbl)
          n749 = call-poly <vilib>:"Ramp Pattern.vi"("start"=w1006, "end"=w1008, "delta"=0.01) -> ("Ramp Pattern"=w1049:dbl[])  [unwired: 6 in, 2 out]
          n750 = call-poly <vilib>:"Ramp Pattern.vi"("start"=w1002, "end"=w1004, "delta"=0.01) -> ("Ramp Pattern"=w1048:dbl[])  [unwired: 6 in, 2 out]
          n751 = local read "Coeff right"() -> (w1047:dbl[])
          n752 = local read "Coeff stop"() -> (w1077:dbl[])
          n753 = local read "Coeff left"() -> (w1098:dbl[])
          n754 = Index Array(array=w1026, index (col) #1=0 ("disabled index (col)")) -> (element #1=w1028:dbl[], element #2=w1030:dbl[])  [unwired: 3 in]
          n755 = Multiply(x=w1045, y=0.5) -> (x*y=w1043:dbl)
          n756 = Multiply(x=w1041, y=0.5) -> (x*y=w1040:dbl)
          n757 = local read "map_track 2"() -> (w1025:dbl[][])
          n758 = call-poly <vilib>:"Polynomial Evaluation.vi"("P(x)"=w1098, "A"=w1049) -> ("P(A)"=w1055:dbl[])  [unwired: 1 out]
          n759 = call-poly <vilib>:"Polynomial Evaluation.vi"("P(x)"=w1047, "A"=w1048) -> ("P(A)"=w1050:dbl[])  [unwired: 1 out]
          n760 = local read "x_shift"() -> (w1019:dbl)
          n761 = call "Convert to Dynamic Data7"("Array"=w1049) -> ("Dynamic Data Type"=w1059:dynamicdata)  [unwired: 3 in]
          n762 = call "Convert to Dynamic Data11"("Array"=w1048) -> ("Dynamic Data Type"=w1058:dynamicdata)  [unwired: 3 in]
          n763 = local read "y_shift"() -> (w1018:dbl)
          n764 = local read "y_end"() -> (w1076:dbl[])
          n765 = call-poly <vilib>:"Ramp Pattern.vi"("start"=w1040, "end"=w1043, "delta"=0.01) -> ("Ramp Pattern"=w1036:dbl[])  [unwired: 6 in, 2 out]
          n766 = global read "G_SEN.vi" "Lane_C_M"() -> (w1039:dbl[])
          n767 = Add(x=w1028, y=w1019) -> (x+y=w1027:dbl[])
          n768 = call-poly <vilib>:"Polynomial Evaluation.vi"("P(x)"=w1077, "A"=w1076) -> ("P(A)"=w1056:dbl[])  [unwired: 1 out]
          n769 = Add(x=w1030, y=w1018) -> (x+y=w1029:dbl[])
          n770 = Build Array(w1055, w1049) -> (w1054:dbl[][])
          n771 = Build Array(w1050, w1048) -> (w1051:dbl[][])
          n772 = call "Convert to Dynamic Data2"("Array"=w1055) -> ("Dynamic Data Type"=w1061:dynamicdata)  [unwired: 3 in]
          n773 = call "Convert to Dynamic Data5"("Array"=w1050) -> ("Dynamic Data Type"=w1060:dynamicdata)  [unwired: 3 in]
          n774 = local read "y 2"() -> (w1097:dbl[])
          n775 = Index Array(array=w1025, index (col) #1=0 ("disabled index (col)")) -> (element #1=w1023:dbl[], element #2=w1021:dbl[])  [unwired: 3 in]
          n776 = local read "y_end"() -> (w1057:dbl[])
          n777 = call-poly <vilib>:"Polynomial Evaluation.vi"("P(x)"=w1039, "A"=w1036) -> ("P(A)"=w1038:dbl[])  [unwired: 1 out]
          n778 = Transpose 2D Array(2D array=w1054) -> (transposed array=w1053:dbl[][])
          n779 = Transpose 2D Array(2D array=w1051) -> (transposed array=w1052:dbl[][])
          n780 = local read "x 2"() -> (w1096:dbl[])
          n781 = call "Convert to Dynamic Data15"("Array"=w1027) -> ("Dynamic Data Type"=w1033:dynamicdata)  [unwired: 3 in]
          n782 = call "Convert to Dynamic Data14"("Array"=w1036) -> ("Dynamic Data Type"=w1035:dynamicdata)  [unwired: 3 in]
          n783 = call "Convert to Dynamic Data17"("Array"=w1023) -> ("Dynamic Data Type"=w1022:dynamicdata)  [unwired: 3 in]
          n784 = call "Convert to Dynamic Data18"("Array"=w1021) -> ("Dynamic Data Type"=w1020:dynamicdata)  [unwired: 3 in]
          n785 = call "Convert to Dynamic Data10"("Array"=w1097) -> ("Dynamic Data Type"=w1068:dynamicdata)  [unwired: 3 in]
          n786 = call "Convert to Dynamic Data"("Array"=w1056) -> ("Dynamic Data Type"=w1066:dynamicdata)  [unwired: 3 in]
          n787 = call "Convert to Dynamic Data16"("Array"=w1029) -> ("Dynamic Data Type"=w1032:dynamicdata)  [unwired: 3 in]
          n788 = call "Convert to Dynamic Data19"() -> ("Dynamic Data Type"=w981:dynamicdata)  [unwired: 4 in]
          n789 = call "Convert to Dynamic Data22"() -> ("Dynamic Data Type"=w978:dynamicdata)  [unwired: 4 in]
          n790 = global write "G_SEN.vi" "Lane_L_V"(w1053) -> ()
          n791 = global write "G_SEN.vi" "Lane_R_V"(w1052) -> ()
          n792 = call "Convert to Dynamic Data9"("Array"=w1096) -> ("Dynamic Data Type"=w1069:dynamicdata)  [unwired: 3 in]
          n793 = call "Convert to Dynamic Data12"("Array"=w1057) -> ("Dynamic Data Type"=w1067:dynamicdata)  [unwired: 3 in]
          n794 = call "Convert to Dynamic Data13"("Array"=w1038) -> ("Dynamic Data Type"=w1037:dynamicdata)  [unwired: 3 in]
          n795 = Merge Signals(w1059, w989, w1058, w986, w1068, w1066, w1035, w1032, w1020, w981, w978) -> (w1070:dynamicdata)
          n796 = call "Convert to Dynamic Data20"() -> ("Dynamic Data Type"=w980:dynamicdata)  [unwired: 4 in]
          n797 = call "Convert to Dynamic Data21"() -> ("Dynamic Data Type"=w979:dynamicdata)  [unwired: 4 in]
          n798 = Merge Signals(w1061, w988, w1060, w987, w1069, w1067, w1037, w1033, w1022, w980, w979) -> (w1071:dynamicdata)
          n799 = call "Build XY Graph"("Y Input"=w1070, "X Input"=w1071) -> ("XY Graph"=→"XY Graph 4":cluster{"X":dbl[], "Y":dbl[]}[])  [unwired: 8 in, 1 out]
        }
        frame Disabled {
        }
      }
    }
  }
